vi "VerifConnection.vi"(8 "error in (no error)":errorcluster, 10 "device connected in":bool, 11 "Sync Box in":refnum<class "Sync Box.lvclass">) -> (0 "error out":errorcluster, 3 "Sync Box out":refnum<class "Sync Box.lvclass">)   [LabVIEW 2018, in "Sync Box.lvclass"]
uses:
  Sync Box.lvclass
  C:/Users/observer/Desktop/Sparc4GUI/SPARC4_GUI/Server/Server.lvclass
  Server/Server.lvclass/Server.ctl
  Server/Server.lvclass
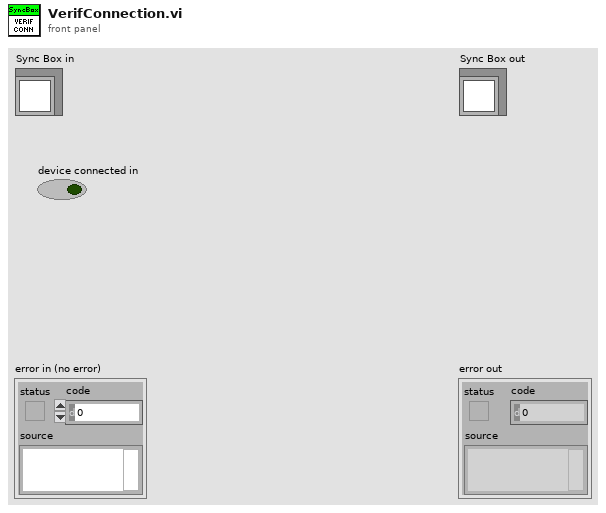
[diagram p1: front panel]
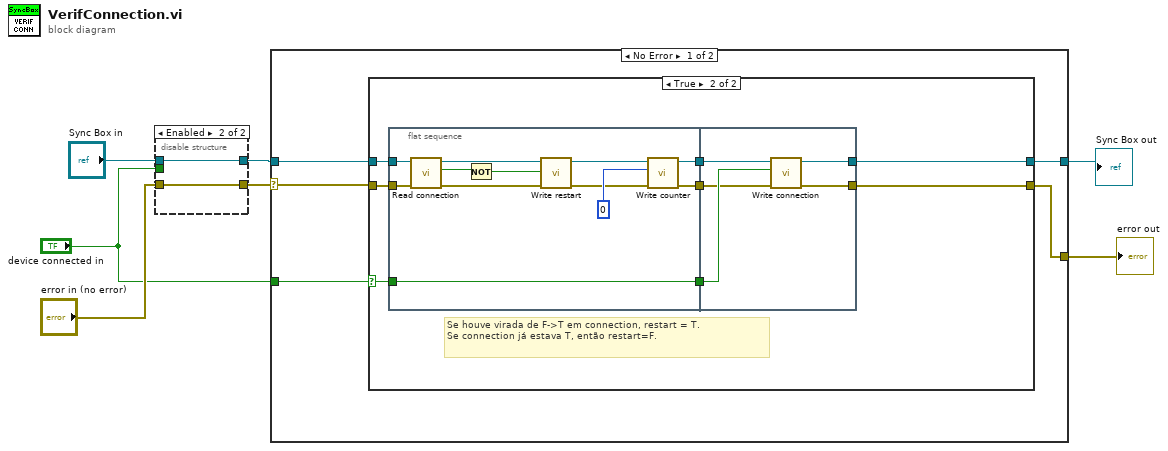
[diagram p0: block diagram]
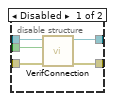
[diagram p2: hidden frame]
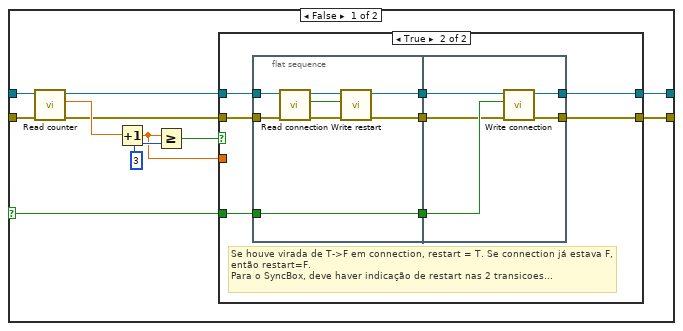
[diagram p3: hidden frame]
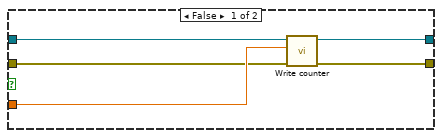
[diagram p4: hidden frame]
diagram:
  n1 = disable-structure shown="Enabled" {
    disable-tunnel: "error in (no error)" -> [w12 w13]
    disable-tunnel: "Sync Box in" -> [w11 w14]
    disable-tunnel: [w10 w14] -> w5
    disable-tunnel: "device connected in" -> [w9 _]
    disable-tunnel: [w8 w13] -> w3
    frame Disabled {
      n2 = call-parent "VerifConnection.vi"("error in (no error)"=w12, "device connected in"=w9, "Server in"=w11) -> ("error out"=w8:errorcluster, "Server out"=w10:refnum<class "Sync Box.lvclass">)  [unwired: 7 in]
    }
    frame Enabled {
    }
  }
  n3 = case shown="No Error" w3 {
    selector: w3 -> [w16 w83]
    tunnel: [w15 w83] -> w1
    tunnel: [w17 w82] -> w2
    tunnel: w5 -> [w19 w82]
    tunnel: "device connected in" -> [w18 _]
    frame No Error {
      n4 = case shown="True" w18 {
        selector: w18 -> [w28 w62]
        tunnel: w19 -> [w25 w64]
        tunnel: [w27 w60] -> w17
        tunnel: w16 -> [w22 w59]
        tunnel: [w20 w57] -> w15
        frame False {
          n5 = call "Read counter.vi"("error in (no error)"=w22, "Server in"=w25) -> ("error out"=w21:errorcluster, "counter"=w23:dbl, "Server out"=w24:refnum<class "Sync Box.lvclass">)  [unwired: 7 in]
          n6 = Increment(x=w23) -> (x+1=w26:dbl)
          n7 = Greater Or Equal?(x=w26, y=u32 3) -> (x >= y?=w29:bool)
          n8 = case shown="True" w29 {
            tunnel: w24 -> [w35 w43]
            tunnel: w28 -> [_ w42]
            tunnel: [w34 w41] -> w27
            tunnel: w26 -> [w33 _]
            tunnel: w21 -> [w32 w37]
            tunnel: [w31 w36] -> w20
            frame False {
              n9 = call "Write counter.vi"("error in (no error)"=w32, "counter"=w33, "Server in"=w35) -> ("error out"=w31:errorcluster, "Server out"=w34:refnum<class "Sync Box.lvclass">)  [unwired: 7 in]
            }
            frame True {
              # "Se houve virada de T->F em connection, restart = T. Se connection já estava F, então restart=F.\nPara o SyncBox, deve haver indicação de restart nas 2 transicoes..."
              n10 = flat-sequence {
                tunnel: w42 -> [w51]
                tunnel: w43 -> [w50]
                tunnel: [w48] -> w40
                tunnel: [w51] -> w39
                tunnel: [w45] -> w38
                tunnel: w37 -> [w44]
                tunnel: [w54] -> w41
                tunnel: w40 -> [w55]
                tunnel: w39 -> [w56]
                tunnel: w38 -> [w53]
                tunnel: [w52] -> w36
                frame #0 {
                  n11 = call "Read connection.vi"("error in (no error)"=w44, "Server in"=w50) -> ("error out"=w47:errorcluster, "connection"=w46:bool, "Server out"=w49:refnum<class "Sync Box.lvclass">)  [unwired: 7 in]
                  n12 = call-dynamic "Write restart.vi"("error in (no error)"=w47, "restart"=w46, "Server in"=w49) -> ("error out"=w45:errorcluster, "Server out"=w48:refnum<class "Sync Box.lvclass">)  [unwired: 7 in]
                }
                frame #1 {
                  n13 = call-dynamic "Write connection.vi"("error in (no error)"=w53, "connection"=w56, "Server in"=w55) -> ("error out"=w52:errorcluster, "Server out"=w54:refnum<class "Sync Box.lvclass">)  [unwired: 7 in]
                }
              }
            }
          }
        }
        frame True {
          # "Se houve virada de F->T em connection, restart = T.\nSe connection já estava T, então restart=F."
          n14 = flat-sequence {
            tunnel: w64 -> [w75]
            tunnel: [w72] -> w63
            tunnel: w62 -> [w76]
            tunnel: [w76] -> w61
            tunnel: w59 -> [w66]
            tunnel: [w65] -> w58
            tunnel: w63 -> [w80]
            tunnel: w61 -> [w81]
            tunnel: [w79] -> w60
            tunnel: w58 -> [w78]
            tunnel: [w77] -> w57
            frame #0 {
              n15 = call "Read connection.vi"("error in (no error)"=w66, "Server in"=w75) -> ("error out"=w69:errorcluster, "connection"=w71:bool, "Server out"=w74:refnum<class "Sync Box.lvclass">)  [unwired: 7 in]
              n16 = Not(x=w71) -> (.not. x?=w70:bool)
              n17 = call-dynamic "Write restart.vi"("error in (no error)"=w69, "restart"=w70, "Server in"=w74) -> ("error out"=w67:errorcluster, "Server out"=w73:refnum<class "Sync Box.lvclass">)  [unwired: 7 in]
              n18 = call "Write counter.vi"("error in (no error)"=w67, "counter"=u32 0, "Server in"=w73) -> ("error out"=w65:errorcluster, "Server out"=w72:refnum<class "Sync Box.lvclass">)  [unwired: 7 in]
            }
            frame #1 {
              n19 = call-dynamic "Write connection.vi"("error in (no error)"=w78, "connection"=w81, "Server in"=w80) -> ("error out"=w77:errorcluster, "Server out"=w79:refnum<class "Sync Box.lvclass">)  [unwired: 7 in]
            }
          }
        }
      }
    }
    frame Error {
    }
  }
  "error out" <- w1
  "Sync Box out" <- w2
